vi "get merge preexisting.vi"(8 "error in (no error)":errorcluster) -> (0 "error out":errorcluster, 3 "function return":bool)   [LabVIEW 2019, in "libSimulationControl.lvlib"]
doc: "bool get_merge_preexisting();"
uses:
  libSimulationControl.lvlib
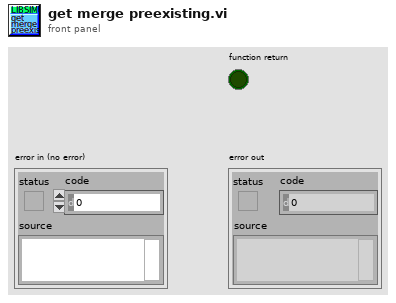
[diagram p1: front panel]
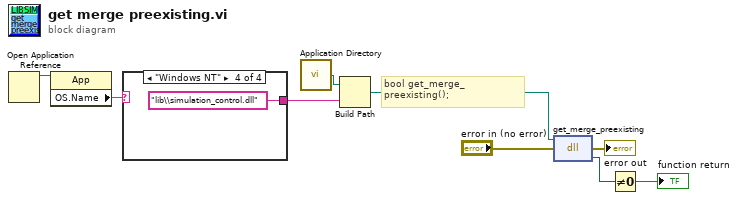
[diagram p0: block diagram]
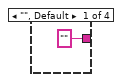
[diagram p2: hidden frame]
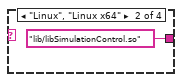
[diagram p3: hidden frame]
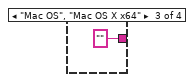
[diagram p4: hidden frame]
diagram:
  # "bool get_merge_preexisting();"
  n1 = Open Application Reference() -> (3:w5:refnum<vi>)  [unwired: 4 in, 1 out]
  n2 = property class="App"(reference=w5) -> ("OS.Name"=w4:string)  [unwired: 1 in, 2 out]
  n3 = case shown="\"Windows NT\"" w4 {
    tunnel: ["" ("return type") "lib/libSimulationControl.so" ("name or relative path") "" ("return type") "lib\\simulation_control.dll" ("name or relative path")] -> w3
    frame "", Default {
    }
    frame "Linux", "Linux x64" {
    }
    frame "Mac OS", "Mac OS X x64" {
    }
    frame "Windows NT" {
    }
  }
  n4 = call <vilib>:"Application Directory.vi"() -> ("Application Directory"=w2:path)
  n5 = Build Path(base path=w2, name or relative path=w3) -> (appended path=w1:path)
  n6 = dll-call lib="home/paul/Schreibtisch/Biogas_plant_setup/LabView/lib/libSimulationControl/libSimulationControl.*" fn="get_merge_preexisting"(path in=w1, error in="error in (no error)") -> (error out=→"error out":errorcluster, "return type"=w8:u8)  [unwired: 1 in, 1 out]
  n7 = Not Equal To 0?(x=w8) -> (x != 0?=→"function return":bool)
